vi "Handle setAllData.vi"(8 "error in (no error)":errorcluster, 10 "AllData":variant, 11 "Instrument.OxfordVRM in":refnum<class "Instrument.OxfordVRM.lvclass">) -> (0 "error out":errorcluster, 3 "Instrument.OxfordVRM out":refnum<class "Instrument.OxfordVRM.lvclass">)   [LabVIEW 2019, in "Instrument.OxfordVRM.lvclass"]
doc: "Override to handle incoming \"setAllData\" command for <b>your</b> Instrument"
uses:
  Instrument.OxfordVRM.lvclass
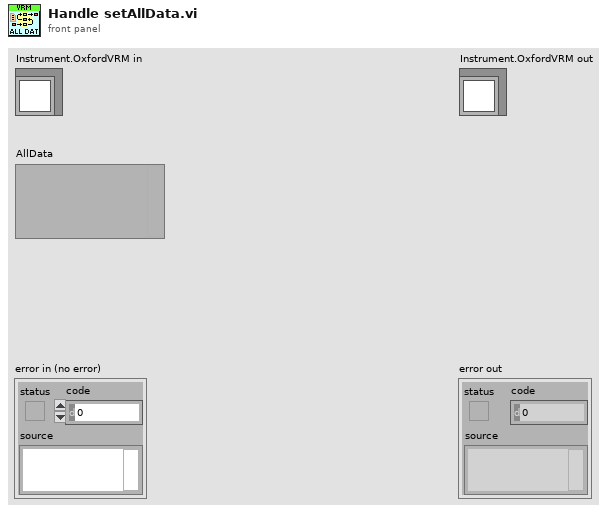
[diagram p1: front panel]
types:
  T1 = typedef "Instrument.OxfordVRM.lvclass/getAll.ctl" = cluster{"Field":dbl[], "Target Field":dbl[], "Target Field Rate":dbl[], "PSU Current":dbl[], "PSU Voltage":dbl[], "Status":string[]}
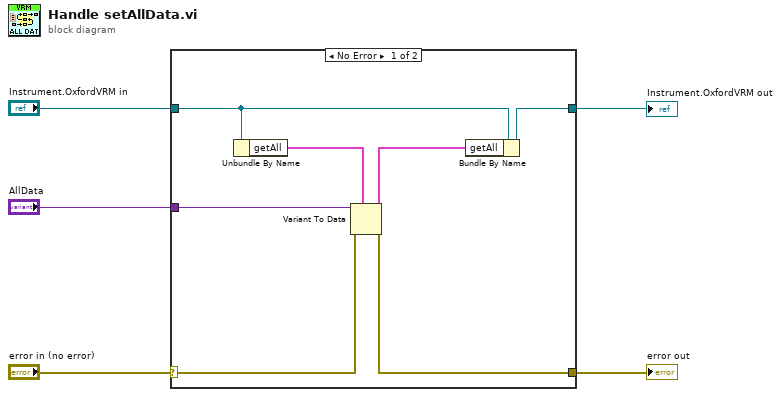
[diagram p0: block diagram]
diagram:
  n1 = case shown="No Error" "error in (no error)" {
    selector: "error in (no error)" -> [w11 w14]
    tunnel: [w10 w14] -> w5
    tunnel: [w6 w13] -> w4
    tunnel: "Instrument.OxfordVRM in" -> [w8 w13]
    tunnel: "AllData" -> [w12 _]
    frame No Error {
      n2 = Unbundle By Name(w8) -> ("getAll"=w9:T1)
      n3 = Variant To Data(error in=w11, type=w9, Variant=w12) -> (data=w7:T1, error out=w10:errorcluster)
      n4 = Bundle By Name(cluster=w8, "getAll"=w7) -> (w6:refnum<class "Instrument.OxfordVRM.lvclass">)
    }
    frame Error {
    }
  }
  "error out" <- w5
  "Instrument.OxfordVRM out" <- w4
